vi "ReadAlgoParametersJSON(Override)_General.vi"(7 "Default?":bool, 8 "error in":errorcluster, 9 "Variant?":bool, 10 "Read Edit Tolerance \nOverride JSON":path=path "F:/User Interface Testbench/Configuration file/Zengage System JSON UI.json", 11 "Algo Default JSON":variant) -> (0 "error out":errorcluster, 2 "data":T1, 3 "Algorithm parameters\noverride":T2)   [LabVIEW 2019, in "ZenGage v3.0 UI.lvclass"]
uses:
  ZenGage v3.0 UI.lvclass
  Type Definitions/JSON Read/Algoparameters_default.ctl
panel:
  out "Error Message":string
  out "VCluster\n out":variant
types:
  T1 = cluster{"AlgoParameters":cluster{"PartsList":cluster{"Name":string, "ImageStreams":cluster{"ThreadName":string, "RackEnable":bool, "ThreadId":dbl, "RackId":dbl, "DifferenceParameter":dbl, "SplitCameraIDs":i32[], "ImagingViews":cluster{"ViewName":string, "ViewEnable":bool, "ImageID":dbl, "CameraID":dbl, "CalibrationFilePath":string, "CalibImageFormat":string, "ReferenceCoordSystem":cluster{"Method":cluster{"Algo":string, "BaseReference":cluster{"OriginX":dbl, "OriginY":dbl, "Angle":dbl, "AxisReference":dbl}}, "ROI":cluster{"ROI":cluster{"Left":dbl, "Top":dbl, "Right":dbl, "Bottom":dbl, "Rotation":dbl}, "EdgeOptions":cluster{"EdgePolarity":dbl, "KernelSize":dbl, "Width":dbl, "MinimumEdgeStrength":dbl, "InterpolationType":dbl, "DataProcessingMethod":dbl}, "LineOptions":cluster{"NumberofLines":dbl, "Type":dbl, "MinScore":dbl, "MaxScore":dbl, "Orientation":dbl, "AngleRange":dbl, "AngleTolerance":dbl, "StepSize":dbl, "MinSNR":dbl, "MinPoints":dbl, "HoughIterations":dbl}, "Process":dbl, "StepSize":dbl, "SearchDirection":dbl, "CircleEdgeOptions":cluster{"SearchDirection":dbl, "EdgeOptions":cluster{"EdgePolarity":dbl, "KernelSize":dbl, "Width":dbl, "MinimumEdgeStrength":dbl, "InterpolationType":dbl, "DataProcessingMethod":dbl}}, "CircleFitOptions":cluster{"Process":dbl, "StepSize":dbl, "MAxPixelRadius":dbl}, "CircleSearchDirection":dbl, "CurveParameters":cluster{"ExtractionMode":dbl, "EdgeThreshold":dbl, "EdgeFilterSize":dbl, "MinLength":dbl, "RowSearchStepSize":dbl, "ColSearchStepSize":dbl, "MaxEndpointGap":dbl, "Closed":bool, "Subpixel":bool}, "MinimumMatchScore":dbl, "CircleDescriptor":cluster{"MinRadius":dbl, "MaxRadius":dbl}, "EllipseDescriptor":cluster{"MinMajorRadius":dbl, "MaxMajorRadius":dbl, "MinMinorRadius":dbl, "MaxMinorRadius":dbl}, "ParallelLines":cluster{"First":dbl, "Second":dbl, "Third":dbl}}[], "Name":string, "OverlayOptions":cluster{"OverlayEnable":bool, "OverlayText":string, "OverlayCoords":i32[], "OverlayAngle":dbl, "OverlayTextSize":dbl, "OverlayTextColor":string, "OverlayROI":bool, "OverlayRakeLine":bool, "OverlayPoints":bool}}, "CameraAngle":i32[]}[]}[], "Measurements":cluster{"RackID":dbl, "ImageID":dbl, "CameraID":dbl, "MeasurementId":dbl, "Name":string, "AlgoName":string, "Type":string, "MeasurementEnable":bool, "AlgorithmSequence":cluster{"RefernceEdge":cluster{"Enable":bool, "Method":string, "RefROI":cluster{"Left":dbl, "Top":dbl, "Right":dbl, "Bottom":dbl, "Rotation":dbl}, "EdgeOptions":cluster{"EdgePoarity":dbl, "KernelSize":dbl, "Width":dbl, "MinimumEdgeStrength":dbl, "InterpolationType":dbl, "DataProcessingMethod":dbl}, "LineOptions":cluster{"NumberofLines":dbl, "Type":dbl, "MinScore":dbl, "MaxScore":dbl, "Orientation":dbl, "AngleRange":dbl, "AngleTolerance":dbl, "StepSize":dbl, "MinSNR":dbl, "MinPoints":dbl, "HoughIterations":dbl}, "SearchDirection":dbl}, "Measurement":cluster{"ROI1":cluster{"Enable":bool, "ROI":cluster{"Left":dbl, "Top":dbl, "Right":dbl, "Bottom":dbl, "Rotation":dbl}, "EdgeOptions":cluster{"EdgePoarity":dbl, "KernelSize":dbl, "Width":dbl, "MinimumEdgeStrength":dbl, "InterpolationType":dbl, "DataProcessingMethod":dbl}, "LineOptions":cluster{"NumberofLines":dbl, "Type":dbl, "MinScore":dbl, "MaxScore":dbl, "Orientation":dbl, "AngleRange":dbl, "AngleTolerance":dbl, "StepSize":dbl, "MinSNR":dbl, "MinPoints":dbl, "HoughIterations":dbl}, "Process":dbl, "StepSize":dbl, "SearchDirection":dbl, "CircleEdgeOptions":cluster{"SearchDirection":dbl, "EdgeOptions":cluster{"EdgePoarity":dbl, "KernelSize":dbl, "Width":dbl, "MinimumEdgeStrength":dbl, "InterpolationType":dbl, "DataProcessingMethod":dbl}}, "CircleFitOptions":cluster{"Process":dbl, "StepSize":dbl, "MAxPixelRadius":dbl}, "CircleSearchDirection":dbl, "CurveParameters":cluster{"ExtractionMode":dbl, "EdgeThreshold":dbl, "EdgeFilterSize":dbl, "MinLength":dbl, "RowSearchStepSize":dbl, "ColSearchStepSize":dbl, "MaxEndpointGap":dbl, "Closed":bool, "Subpixel":bool}, "MinimumMatchScore":dbl, "CircleDescriptor":cluster{"MinRadius":dbl, "MaxRadius":dbl}, "EllipseDescriptor":cluster{"MinMajorRadius":dbl, "MaxMajorRadius":dbl, "MinMinorRadius":dbl, "MaxMinorRadius":dbl}}, "ROI2":cluster{"Enable":bool, "ROI":cluster{"Left":dbl, "Top":dbl, "Right":dbl, "Bottom":dbl, "Rotation":dbl}, "EdgeOptions":cluster{"EdgePoarity":dbl, "KernelSize":dbl, "Width":dbl, "MinimumEdgeStrength":dbl, "InterpolationType":dbl, "DataProcessingMethod":dbl}, "LineOptions":cluster{"NumberofLines":dbl, "Type":dbl, "MinScore":dbl, "MaxScore":dbl, "Orientation":dbl, "AngleRange":dbl, "AngleTolerance":dbl, "StepSize":dbl, "MinSNR":dbl, "MinPoints":dbl, "HoughIterations":dbl}, "Process":dbl, "StepSize":dbl, "SearchDirection":dbl, "CircleEdgeOptions":cluster{"SearchDirection":dbl, "EdgeOptions":cluster{"EdgePoarity":dbl, "KernelSize":dbl, "Width":dbl, "MinimumEdgeStrength":dbl, "InterpolationType":dbl, "DataProcessingMethod":dbl}}, "CircleFitOptions":cluster{"Process":dbl, "StepSize":dbl, "MAxPixelRadius":dbl}, "CircleSearchDirection":dbl, "CurveParameters":cluster{"ExtractionMode":dbl, "EdgeThreshold":dbl, "EdgeFilterSize":dbl, "MinLength":dbl, "RowSearchStepSize":dbl, "ColSearchStepSize":dbl, "MaxEndpointGap":dbl, "Closed":bool, "Subpixel":bool}, "MinimumMatchScore":dbl, "CircleDescriptor":cluster{"MinRadius":dbl, "MaxRadius":dbl}, "EllipseDescriptor":cluster{"MinMajorRadius":dbl, "MaxMajorRadius":dbl, "MinMinorRadius":dbl, "MaxMinorRadius":dbl}}}}, "MathExpression":cluster{"Algorithm":string, "MathExpression":string, "ResultVariable":string}, "MathCorrectionParameters":cluster{"Radius":dbl, "CurlGap":dbl, "Thickness":dbl, "MeasurementIndices":i32[], "MathAlgoName":string, "MathAlgoFormula":string, "CorrectionForAngle":i32[], "NumericAray":i32[], "StringArray":string[]}, "ResultVariableCluster":cluster{"RVName":string, "RVSequence":string, "RVIndex":dbl, "RVID":dbl, "RVValue":dbl}, "CalibrationCoefficients":cluster{"A1":dbl, "A2":dbl, "A3":dbl}, "UserCalibCoefficients":cluster{"UserCorrectionLinearityCoeff":dbl, "UserCorrectionBiasCoeff":dbl}, "SpecValues":cluster{"LCL":dbl, "UCL":dbl, "LSL":dbl, "USL":dbl, "NominalValue":dbl}, "OverlayOptions":cluster{"OverlayEnable":bool, "OverlayText":string, "OverlayCoords":i32[], "OverlayAngle":dbl, "OverlayTextSize":dbl, "OverlayTextColor":string, "OverlayROI":bool, "OverlayRakeLine":bool, "OverlayPoints":bool}, "DatalogEnable":bool, "DisplayIcon":string}[]}[], "AlgoDefaultParameters":cluster{"AlgoName":string, "Enable":bool, "AlgorithmSequenceDefault":cluster{"RefernceEdgeDefault":cluster{"Method":string, "RefROI":cluster{"Left":dbl, "Top":dbl, "Right":dbl, "Bottom":dbl, "Rotation":dbl}, "EdgeOptions":cluster{"EdgePoarity":dbl, "KernelSize":dbl, "Width":dbl, "MinimumEdgeStrength":dbl, "InterpolationType":dbl, "DataProcessingMethod":dbl}, "LineOptions":cluster{"NumberofLines":dbl, "Type":dbl, "MinScore":dbl, "MaxScore":dbl, "Orientation":dbl, "AngleRange":dbl, "AngleTolerance":dbl, "StepSize":dbl, "MinSNR":dbl, "MinPoints":dbl, "HoughIterations":dbl}, "SearchDirection":dbl}, "MeasurementDefault":cluster{"ROI1":cluster{"ROI":cluster{"Left":dbl, "Top":dbl, "Right":dbl, "Bottom":dbl, "Rotation":dbl}, "EdgeOptions":cluster{"EdgePoarity":dbl, "KernelSize":dbl, "Width":dbl, "MinimumEdgeStrength":dbl, "InterpolationType":dbl, "DataProcessingMethod":dbl}, "LineOptions":cluster{"NumberofLines":dbl, "Type":dbl, "MinScore":dbl, "MaxScore":dbl, "Orientation":dbl, "AngleRange":dbl, "AngleTolerance":dbl, "StepSize":dbl, "MinSNR":dbl, "MinPoints":dbl, "HoughIterations":dbl}, "Process":dbl, "StepSize":dbl, "SearchDirection":dbl, "CircleEdgeOptions":cluster{"SearchDirection":dbl, "EdgeOptions":cluster{"EdgePoarity":dbl, "KernelSize":dbl, "Width":dbl, "MinimumEdgeStrength":dbl, "InterpolationType":dbl, "DataProcessingMethod":dbl}}, "CircleFitOptions":cluster{"Process":dbl, "StepSize":dbl, "MAxPixelRadius":dbl}, "CircleSearchDirection":dbl, "CurveParameters":cluster{"ExtractionMode":dbl, "EdgeThreshold":dbl, "EdgeFilterSize":dbl, "MinLength":dbl, "RowSearchStepSize":dbl, "ColSearchStepSize":dbl, "MaxEndpointGap":dbl, "Closed":dbl, "Subpixel":dbl}, "MinimumMatchScore":dbl, "CircleDescriptor":cluster{"MinRadius":dbl, "MaxRadius":dbl}, "EllipseDescriptor":cluster{"MinMajorRadius":dbl, "MaxMajorRadius":dbl, "MinMinorRadius":dbl, "MaxMinorRadius":dbl}, "OverlayOptions":cluster{"OverlayEnable":bool, "OverlayText":string, "OverlayCoords":i32[], "OverlayAngle":dbl, "OverlayTextSize":dbl, "OverlayTextColor":string}, "ResultVariable":string}, "ROI2":cluster{"ROI":cluster{"Left":dbl, "Top":dbl, "Right":dbl, "Bottom":dbl, "Rotation":dbl}, "EdgeOptions":cluster{"EdgePoarity":dbl, "KernelSize":dbl, "Width":dbl, "MinimumEdgeStrength":dbl, "InterpolationType":dbl, "DataProcessingMethod":dbl}, "LineOptions":cluster{"NumberofLines":dbl, "Type":dbl, "MinScore":dbl, "MaxScore":dbl, "Orientation":dbl, "AngleRange":dbl, "AngleTolerance":dbl, "StepSize":dbl, "MinSNR":dbl, "MinPoints":dbl, "HoughIterations":dbl}, "Process":dbl, "StepSize":dbl, "SearchDirection":dbl, "CircleEdgeOptions":cluster{"SearchDirection":dbl, "EdgeOptions":cluster{"EdgePoarity":dbl, "KernelSize":dbl, "Width":dbl, "MinimumEdgeStrength":dbl, "InterpolationType":dbl, "DataProcessingMethod":dbl}}, "CircleFitOptions":cluster{"Process":dbl, "StepSize":dbl, "MaxPixelRadius":dbl}, "CircleSearchDirection":dbl, "CurveParameters":cluster{"ExtractionMode":dbl, "EdgeThreshold":dbl, "EdgeFilterSize":dbl, "MinLength":dbl, "RowSearchStepSize":dbl, "ColSearchStepSize":dbl, "MaxEndpointGap":dbl, "Closed":dbl, "Subpixel":dbl}, "MinimumMatchScore":dbl, "CircleDescriptor":cluster{"MinRadius":dbl, "MaxRadius":dbl}, "EllipseDescriptor":cluster{"MinMajorRadius":dbl, "MaxMajorRadius":dbl, "MinMinorRadius":dbl, "MaxMinorRadius":dbl}, "OverlayOptions":cluster{"OverlayEnable":bool, "OverlayText":string, "OverlayCoords":i32[], "OverlayAngle":dbl, "OverlayTextSize":dbl, "OverlayTextColor":string}, "ResultVariable":string}}, "MathExpressionDefault":cluster{"Algorithm":string, "MathExpression":string, "ResultVariable":string}}, "CalibrationCoefficients":cluster{"A1":dbl, "A2":dbl, "A3":dbl}, "UserCalibCoefficients":cluster{"UserCorrectionBiasCoeff":dbl, "UserCorrectionLinearityCoeff":dbl}, "OverlayOptions":cluster{"OverlayEnable":bool, "OverlayText":string, "OverlayCoords":i32[], "OverlayAngle":dbl, "OverlayTextSize":dbl, "OverlayTextColor":string}, "DatalogEnable":bool, "DisplayIcon":string}}}
  T2 = typedef "ZenGage v3.0 UI.lvclass/Algoparameters_default.ctl" = cluster{"AlgoParameters":cluster{"PartsList":cluster{"Name":string, "ImageStreams":cluster{"ThreadName":string, "RackEnable":bool, "ThreadId":dbl, "RackId":dbl, "DifferenceParameter":dbl, "SplitCameraIDs":i32[], "ImagingViews":cluster{"ViewName":string, "ViewEnable":bool, "ImageID":dbl, "CameraID":dbl, "CalibrationFilePath":string, "CalibImageFormat":string, "ReferenceCoordSystem":cluster{"Method":cluster{"Algo":string, "BaseReference":cluster{"OriginX":dbl, "OriginY":dbl, "Angle":dbl, "AxisReference":dbl}}, "ROI":cluster{"ROI":cluster{"Left":dbl, "Top":dbl, "Right":dbl, "Bottom":dbl, "Rotation":dbl}, "EdgeOptions":cluster{"EdgePolarity":dbl, "KernelSize":dbl, "Width":dbl, "MinimumEdgeStrength":dbl, "InterpolationType":dbl, "DataProcessingMethod":dbl}, "LineOptions":cluster{"NumberofLines":dbl, "Type":dbl, "MinScore":dbl, "MaxScore":dbl, "Orientation":dbl, "AngleRange":dbl, "AngleTolerance":dbl, "StepSize":dbl, "MinSNR":dbl, "MinPoints":dbl, "HoughIterations":dbl}, "Process":dbl, "StepSize":dbl, "SearchDirection":dbl, "CircleEdgeOptions":cluster{"SearchDirection":dbl, "EdgeOptions":cluster{"EdgePolarity":dbl, "KernelSize":dbl, "Width":dbl, "MinimumEdgeStrength":dbl, "InterpolationType":dbl, "DataProcessingMethod":dbl}}, "CircleFitOptions":cluster{"Process":dbl, "StepSize":dbl, "MAxPixelRadius":dbl}, "CircleSearchDirection":dbl, "CurveParameters":cluster{"ExtractionMode":dbl, "EdgeThreshold":dbl, "EdgeFilterSize":dbl, "MinLength":dbl, "RowSearchStepSize":dbl, "ColSearchStepSize":dbl, "MaxEndpointGap":dbl, "Closed":bool, "Subpixel":bool}, "MinimumMatchScore":dbl, "CircleDescriptor":cluster{"MinRadius":dbl, "MaxRadius":dbl}, "EllipseDescriptor":cluster{"MinMajorRadius":dbl, "MaxMajorRadius":dbl, "MinMinorRadius":dbl, "MaxMinorRadius":dbl}, "ParallelLines":cluster{"First":dbl, "Second":dbl, "Third":dbl}}[], "Name":string, "OverlayOptions":cluster{"OverlayEnable":bool, "OverlayText":string, "OverlayCoords":i32[], "OverlayAngle":dbl, "OverlayTextSize":dbl, "OverlayTextColor":string, "OverlayROI":bool, "OverlayRakeLine":bool, "OverlayPoints":bool}}}[]}[], "Measurements":cluster{"RackID":dbl, "ImageID":dbl, "CameraID":dbl, "MeasurementId":dbl, "Name":string, "AlgoName":string, "Type":string, "MeasurementEnable":bool, "AlgorithmSequence":cluster{"RefernceEdge":cluster{"Enable":bool, "Method":string, "RefROI":cluster{"Left":dbl, "Top":dbl, "Right":dbl, "Bottom":dbl, "Rotation":dbl}, "EdgeOptions":cluster{"EdgePoarity":dbl, "KernelSize":dbl, "Width":dbl, "MinimumEdgeStrength":dbl, "InterpolationType":dbl, "DataProcessingMethod":dbl}, "LineOptions":cluster{"NumberofLines":dbl, "Type":dbl, "MinScore":dbl, "MaxScore":dbl, "Orientation":dbl, "AngleRange":dbl, "AngleTolerance":dbl, "StepSize":dbl, "MinSNR":dbl, "MinPoints":dbl, "HoughIterations":dbl}, "SearchDirection":dbl}, "Measurement":cluster{"ROI1":cluster{"Enable":bool, "ROI":cluster{"Left":dbl, "Top":dbl, "Right":dbl, "Bottom":dbl, "Rotation":dbl}, "EdgeOptions":cluster{"EdgePoarity":dbl, "KernelSize":dbl, "Width":dbl, "MinimumEdgeStrength":dbl, "InterpolationType":dbl, "DataProcessingMethod":dbl}, "LineOptions":cluster{"NumberofLines":dbl, "Type":dbl, "MinScore":dbl, "MaxScore":dbl, "Orientation":dbl, "AngleRange":dbl, "AngleTolerance":dbl, "StepSize":dbl, "MinSNR":dbl, "MinPoints":dbl, "HoughIterations":dbl}, "Process":dbl, "StepSize":dbl, "SearchDirection":dbl, "CircleEdgeOptions":cluster{"SearchDirection":dbl, "EdgeOptions":cluster{"EdgePoarity":dbl, "KernelSize":dbl, "Width":dbl, "MinimumEdgeStrength":dbl, "InterpolationType":dbl, "DataProcessingMethod":dbl}}, "CircleFitOptions":cluster{"Process":dbl, "StepSize":dbl, "MAxPixelRadius":dbl}, "CircleSearchDirection":dbl, "CurveParameters":cluster{"ExtractionMode":dbl, "EdgeThreshold":dbl, "EdgeFilterSize":dbl, "MinLength":dbl, "RowSearchStepSize":dbl, "ColSearchStepSize":dbl, "MaxEndpointGap":dbl, "Closed":bool, "Subpixel":bool}, "MinimumMatchScore":dbl, "CircleDescriptor":cluster{"MinRadius":dbl, "MaxRadius":dbl}, "EllipseDescriptor":cluster{"MinMajorRadius":dbl, "MaxMajorRadius":dbl, "MinMinorRadius":dbl, "MaxMinorRadius":dbl}}, "ROI2":cluster{"Enable":bool, "ROI":cluster{"Left":dbl, "Top":dbl, "Right":dbl, "Bottom":dbl, "Rotation":dbl}, "EdgeOptions":cluster{"EdgePoarity":dbl, "KernelSize":dbl, "Width":dbl, "MinimumEdgeStrength":dbl, "InterpolationType":dbl, "DataProcessingMethod":dbl}, "LineOptions":cluster{"NumberofLines":dbl, "Type":dbl, "MinScore":dbl, "MaxScore":dbl, "Orientation":dbl, "AngleRange":dbl, "AngleTolerance":dbl, "StepSize":dbl, "MinSNR":dbl, "MinPoints":dbl, "HoughIterations":dbl}, "Process":dbl, "StepSize":dbl, "SearchDirection":dbl, "CircleEdgeOptions":cluster{"SearchDirection":dbl, "EdgeOptions":cluster{"EdgePoarity":dbl, "KernelSize":dbl, "Width":dbl, "MinimumEdgeStrength":dbl, "InterpolationType":dbl, "DataProcessingMethod":dbl}}, "CircleFitOptions":cluster{"Process":dbl, "StepSize":dbl, "MAxPixelRadius":dbl}, "CircleSearchDirection":dbl, "CurveParameters":cluster{"ExtractionMode":dbl, "EdgeThreshold":dbl, "EdgeFilterSize":dbl, "MinLength":dbl, "RowSearchStepSize":dbl, "ColSearchStepSize":dbl, "MaxEndpointGap":dbl, "Closed":bool, "Subpixel":bool}, "MinimumMatchScore":dbl, "CircleDescriptor":cluster{"MinRadius":dbl, "MaxRadius":dbl}, "EllipseDescriptor":cluster{"MinMajorRadius":dbl, "MaxMajorRadius":dbl, "MinMinorRadius":dbl, "MaxMinorRadius":dbl}}}}, "MathExpression":cluster{"Algorithm":string, "MathExpression":string, "ResultVariable":string}, "ResultVariableCluster":cluster{"RVName":string, "RVSequence":string, "RVIndex":dbl, "RVID":dbl, "RVValue":dbl}, "CalibrationCoefficients":cluster{"A1":dbl, "A2":dbl, "A3":dbl}, "UserCalibCoefficients":cluster{"UserCorrectionLinearityCoeff":dbl, "UserCorrectionBiasCoeff":dbl}, "SpecValues":cluster{"LCL":dbl, "UCL":dbl, "LSL":dbl, "USL":dbl, "NominalValue":dbl}, "OverlayOptions":cluster{"OverlayEnable":bool, "OverlayText":string, "OverlayCoords":i32[], "OverlayAngle":dbl, "OverlayTextSize":dbl, "OverlayTextColor":string, "OverlayROI":bool, "OverlayRakeLine":bool, "OverlayPoints":bool}, "DatalogEnable":bool, "DisplayIcon":string}[]}[], "AlgoDefaultParameters":cluster{"AlgoName":string, "Enable":bool, "AlgorithmSequenceDefault":cluster{"RefernceEdgeDefault":cluster{"Method":string, "RefROI":cluster{"Left":dbl, "Top":dbl, "Right":dbl, "Bottom":dbl, "Rotation":dbl}, "EdgeOptions":cluster{"EdgePoarity":dbl, "KernelSize":dbl, "Width":dbl, "MinimumEdgeStrength":dbl, "InterpolationType":dbl, "DataProcessingMethod":dbl}, "LineOptions":cluster{"NumberofLines":dbl, "Type":dbl, "MinScore":dbl, "MaxScore":dbl, "Orientation":dbl, "AngleRange":dbl, "AngleTolerance":dbl, "StepSize":dbl, "MinSNR":dbl, "MinPoints":dbl, "HoughIterations":dbl}, "SearchDirection":dbl}, "MeasurementDefault":cluster{"ROI1":cluster{"ROI":cluster{"Left":dbl, "Top":dbl, "Right":dbl, "Bottom":dbl, "Rotation":dbl}, "EdgeOptions":cluster{"EdgePoarity":dbl, "KernelSize":dbl, "Width":dbl, "MinimumEdgeStrength":dbl, "InterpolationType":dbl, "DataProcessingMethod":dbl}, "LineOptions":cluster{"NumberofLines":dbl, "Type":dbl, "MinScore":dbl, "MaxScore":dbl, "Orientation":dbl, "AngleRange":dbl, "AngleTolerance":dbl, "StepSize":dbl, "MinSNR":dbl, "MinPoints":dbl, "HoughIterations":dbl}, "Process":dbl, "StepSize":dbl, "SearchDirection":dbl, "CircleEdgeOptions":cluster{"SearchDirection":dbl, "EdgeOptions":cluster{"EdgePoarity":dbl, "KernelSize":dbl, "Width":dbl, "MinimumEdgeStrength":dbl, "InterpolationType":dbl, "DataProcessingMethod":dbl}}, "CircleFitOptions":cluster{"Process":dbl, "StepSize":dbl, "MAxPixelRadius":dbl}, "CircleSearchDirection":dbl, "CurveParameters":cluster{"ExtractionMode":dbl, "EdgeThreshold":dbl, "EdgeFilterSize":dbl, "MinLength":dbl, "RowSearchStepSize":dbl, "ColSearchStepSize":dbl, "MaxEndpointGap":dbl, "Closed":dbl, "Subpixel":dbl}, "MinimumMatchScore":dbl, "CircleDescriptor":cluster{"MinRadius":dbl, "MaxRadius":dbl}, "EllipseDescriptor":cluster{"MinMajorRadius":dbl, "MaxMajorRadius":dbl, "MinMinorRadius":dbl, "MaxMinorRadius":dbl}, "OverlayOptions":cluster{"OverlayEnable":bool, "OverlayText":string, "OverlayCoords":i32[], "OverlayAngle":dbl, "OverlayTextSize":dbl, "OverlayTextColor":string}, "ResultVariable":string}, "ROI2":cluster{"ROI":cluster{"Left":dbl, "Top":dbl, "Right":dbl, "Bottom":dbl, "Rotation":dbl}, "EdgeOptions":cluster{"EdgePoarity":dbl, "KernelSize":dbl, "Width":dbl, "MinimumEdgeStrength":dbl, "InterpolationType":dbl, "DataProcessingMethod":dbl}, "LineOptions":cluster{"NumberofLines":dbl, "Type":dbl, "MinScore":dbl, "MaxScore":dbl, "Orientation":dbl, "AngleRange":dbl, "AngleTolerance":dbl, "StepSize":dbl, "MinSNR":dbl, "MinPoints":dbl, "HoughIterations":dbl}, "Process":dbl, "StepSize":dbl, "SearchDirection":dbl, "CircleEdgeOptions":cluster{"SearchDirection":dbl, "EdgeOptions":cluster{"EdgePoarity":dbl, "KernelSize":dbl, "Width":dbl, "MinimumEdgeStrength":dbl, "InterpolationType":dbl, "DataProcessingMethod":dbl}}, "CircleFitOptions":cluster{"Process":dbl, "StepSize":dbl, "MaxPixelRadius":dbl}, "CircleSearchDirection":dbl, "CurveParameters":cluster{"ExtractionMode":dbl, "EdgeThreshold":dbl, "EdgeFilterSize":dbl, "MinLength":dbl, "RowSearchStepSize":dbl, "ColSearchStepSize":dbl, "MaxEndpointGap":dbl, "Closed":dbl, "Subpixel":dbl}, "MinimumMatchScore":dbl, "CircleDescriptor":cluster{"MinRadius":dbl, "MaxRadius":dbl}, "EllipseDescriptor":cluster{"MinMajorRadius":dbl, "MaxMajorRadius":dbl, "MinMinorRadius":dbl, "MaxMinorRadius":dbl}, "OverlayOptions":cluster{"OverlayEnable":bool, "OverlayText":string, "OverlayCoords":i32[], "OverlayAngle":dbl, "OverlayTextSize":dbl, "OverlayTextColor":string}, "ResultVariable":string}}, "MathExpressionDefault":cluster{"Algorithm":string, "MathExpression":string, "ResultVariable":string}}, "CalibrationCoefficients":cluster{"A1":dbl, "A2":dbl, "A3":dbl}, "UserCalibCoefficients":cluster{"UserCorrectionBiasCoeff":dbl, "UserCorrectionLinearityCoeff":dbl}, "OverlayOptions":cluster{"OverlayEnable":bool, "OverlayText":string, "OverlayCoords":i32[], "OverlayAngle":dbl, "OverlayTextSize":dbl, "OverlayTextColor":string}, "DatalogEnable":bool, "DisplayIcon":string}}}
  T3 = cluster{"SpecificationVersion":string, "CompatibleSoftwareVersions":string[], "AlgoParameters":cluster{"PartsList":cluster{"Name":string, "ImageStreams":cluster{"ThreadName":string, "RackEnable":bool, "ThreadId":dbl, "RackId":dbl, "DifferenceParameter":dbl, "SplitCameraIDs":i32[], "ImagingViews":cluster{"ViewName":string, "ViewEnable":bool, "ImageID":dbl, "CameraID":dbl, "CalibrationFilePath":string, "CalibImageFormat":string, "ReferenceCoordSystem":cluster{"Method":cluster{"Algo":string, "BaseReference":cluster{"OriginX":dbl, "OriginY":dbl, "Angle":dbl, "AxisReference":dbl}}, "ROI":cluster{"ROI":cluster{"Left":dbl, "Top":dbl, "Right":dbl, "Bottom":dbl, "Rotation":dbl}, "EdgeOptions":cluster{"EdgePolarity":dbl, "KernelSize":dbl, "Width":dbl, "MinimumEdgeStrength":dbl, "InterpolationType":dbl, "DataProcessingMethod":dbl}, "LineOptions":cluster{"NumberofLines":dbl, "Type":dbl, "MinScore":dbl, "MaxScore":dbl, "Orientation":dbl, "AngleRange":dbl, "AngleTolerance":dbl, "StepSize":dbl, "MinSNR":dbl, "MinPoints":dbl, "HoughIterations":dbl}, "Process":dbl, "StepSize":dbl, "SearchDirection":dbl, "CircleEdgeOptions":cluster{"SearchDirection":dbl, "EdgeOptions":cluster{"EdgePolarity":dbl, "KernelSize":dbl, "Width":dbl, "MinimumEdgeStrength":dbl, "InterpolationType":dbl, "DataProcessingMethod":dbl}}, "CircleFitOptions":cluster{"Process":dbl, "StepSize":dbl, "MAxPixelRadius":dbl}, "CircleSearchDirection":dbl, "CurveParameters":cluster{"ExtractionMode":dbl, "EdgeThreshold":dbl, "EdgeFilterSize":dbl, "MinLength":dbl, "RowSearchStepSize":dbl, "ColSearchStepSize":dbl, "MaxEndpointGap":dbl, "Closed":bool, "Subpixel":bool}, "MinimumMatchScore":dbl, "CircleDescriptor":cluster{"MinRadius":dbl, "MaxRadius":dbl}, "EllipseDescriptor":cluster{"MinMajorRadius":dbl, "MaxMajorRadius":dbl, "MinMinorRadius":dbl, "MaxMinorRadius":dbl}, "ParallelLines":cluster{"First":dbl, "Second":dbl, "Third":dbl}}[], "Name":string, "OverlayOptions":cluster{"OverlayEnable":bool, "OverlayText":string, "OverlayCoords":i32[], "OverlayAngle":dbl, "OverlayTextSize":dbl, "OverlayTextColor":string, "OverlayROI":bool, "OverlayRakeLine":bool, "OverlayPoints":bool}}, "CameraAngle":i32[]}[]}[], "Measurements":cluster{"RackID":dbl, "ImageID":dbl, "CameraID":dbl, "MeasurementId":dbl, "Name":string, "AlgoName":string, "Type":string, "MeasurementEnable":bool, "AlgorithmSequence":cluster{"RefernceEdge":cluster{"Enable":bool, "Method":string, "RefROI":cluster{"Left":dbl, "Top":dbl, "Right":dbl, "Bottom":dbl, "Rotation":dbl}, "EdgeOptions":cluster{"EdgePoarity":dbl, "KernelSize":dbl, "Width":dbl, "MinimumEdgeStrength":dbl, "InterpolationType":dbl, "DataProcessingMethod":dbl}, "LineOptions":cluster{"NumberofLines":dbl, "Type":dbl, "MinScore":dbl, "MaxScore":dbl, "Orientation":dbl, "AngleRange":dbl, "AngleTolerance":dbl, "StepSize":dbl, "MinSNR":dbl, "MinPoints":dbl, "HoughIterations":dbl}, "SearchDirection":dbl}, "Measurement":cluster{"ROI1":cluster{"Enable":bool, "ROI":cluster{"Left":dbl, "Top":dbl, "Right":dbl, "Bottom":dbl, "Rotation":dbl}, "EdgeOptions":cluster{"EdgePoarity":dbl, "KernelSize":dbl, "Width":dbl, "MinimumEdgeStrength":dbl, "InterpolationType":dbl, "DataProcessingMethod":dbl}, "LineOptions":cluster{"NumberofLines":dbl, "Type":dbl, "MinScore":dbl, "MaxScore":dbl, "Orientation":dbl, "AngleRange":dbl, "AngleTolerance":dbl, "StepSize":dbl, "MinSNR":dbl, "MinPoints":dbl, "HoughIterations":dbl}, "Process":dbl, "StepSize":dbl, "SearchDirection":dbl, "CircleEdgeOptions":cluster{"SearchDirection":dbl, "EdgeOptions":cluster{"EdgePoarity":dbl, "KernelSize":dbl, "Width":dbl, "MinimumEdgeStrength":dbl, "InterpolationType":dbl, "DataProcessingMethod":dbl}}, "CircleFitOptions":cluster{"Process":dbl, "StepSize":dbl, "MAxPixelRadius":dbl}, "CircleSearchDirection":dbl, "CurveParameters":cluster{"ExtractionMode":dbl, "EdgeThreshold":dbl, "EdgeFilterSize":dbl, "MinLength":dbl, "RowSearchStepSize":dbl, "ColSearchStepSize":dbl, "MaxEndpointGap":dbl, "Closed":bool, "Subpixel":bool}, "MinimumMatchScore":dbl, "CircleDescriptor":cluster{"MinRadius":dbl, "MaxRadius":dbl}, "EllipseDescriptor":cluster{"MinMajorRadius":dbl, "MaxMajorRadius":dbl, "MinMinorRadius":dbl, "MaxMinorRadius":dbl}}, "ROI2":cluster{"Enable":bool, "ROI":cluster{"Left":dbl, "Top":dbl, "Right":dbl, "Bottom":dbl, "Rotation":dbl}, "EdgeOptions":cluster{"EdgePoarity":dbl, "KernelSize":dbl, "Width":dbl, "MinimumEdgeStrength":dbl, "InterpolationType":dbl, "DataProcessingMethod":dbl}, "LineOptions":cluster{"NumberofLines":dbl, "Type":dbl, "MinScore":dbl, "MaxScore":dbl, "Orientation":dbl, "AngleRange":dbl, "AngleTolerance":dbl, "StepSize":dbl, "MinSNR":dbl, "MinPoints":dbl, "HoughIterations":dbl}, "Process":dbl, "StepSize":dbl, "SearchDirection":dbl, "CircleEdgeOptions":cluster{"SearchDirection":dbl, "EdgeOptions":cluster{"EdgePoarity":dbl, "KernelSize":dbl, "Width":dbl, "MinimumEdgeStrength":dbl, "InterpolationType":dbl, "DataProcessingMethod":dbl}}, "CircleFitOptions":cluster{"Process":dbl, "StepSize":dbl, "MAxPixelRadius":dbl}, "CircleSearchDirection":dbl, "CurveParameters":cluster{"ExtractionMode":dbl, "EdgeThreshold":dbl, "EdgeFilterSize":dbl, "MinLength":dbl, "RowSearchStepSize":dbl, "ColSearchStepSize":dbl, "MaxEndpointGap":dbl, "Closed":bool, "Subpixel":bool}, "MinimumMatchScore":dbl, "CircleDescriptor":cluster{"MinRadius":dbl, "MaxRadius":dbl}, "EllipseDescriptor":cluster{"MinMajorRadius":dbl, "MaxMajorRadius":dbl, "MinMinorRadius":dbl, "MaxMinorRadius":dbl}}}}, "MathExpression":cluster{"Algorithm":string, "MathExpression":string, "ResultVariable":string}, "MathCorrectionParameters":cluster{"Radius":dbl, "CurlGap":dbl, "Thickness":dbl, "MeasurementIndices":i32[], "MathAlgoName":string, "MathAlgoFormula":string, "CorrectionForAngle":i32[], "NumericAray":i32[], "StringArray":string[]}, "ResultVariableCluster":cluster{"RVName":string, "RVSequence":string, "RVIndex":dbl, "RVID":dbl, "RVValue":dbl}, "CalibrationCoefficients":cluster{"A1":dbl, "A2":dbl, "A3":dbl}, "UserCalibCoefficients":cluster{"UserCorrectionLinearityCoeff":dbl, "UserCorrectionBiasCoeff":dbl}, "SpecValues":cluster{"LCL":dbl, "UCL":dbl, "LSL":dbl, "USL":dbl, "NominalValue":dbl}, "OverlayOptions":cluster{"OverlayEnable":bool, "OverlayText":string, "OverlayCoords":i32[], "OverlayAngle":dbl, "OverlayTextSize":dbl, "OverlayTextColor":string, "OverlayROI":bool, "OverlayRakeLine":bool, "OverlayPoints":bool}, "DatalogEnable":bool, "DisplayIcon":string}[]}[], "AlgoDefaultParameters":cluster{"AlgoName":string, "Enable":bool, "AlgorithmSequenceDefault":cluster{"RefernceEdgeDefault":cluster{"Method":string, "RefROI":cluster{"Left":dbl, "Top":dbl, "Right":dbl, "Bottom":dbl, "Rotation":dbl}, "EdgeOptions":cluster{"EdgePoarity":dbl, "KernelSize":dbl, "Width":dbl, "MinimumEdgeStrength":dbl, "InterpolationType":dbl, "DataProcessingMethod":dbl}, "LineOptions":cluster{"NumberofLines":dbl, "Type":dbl, "MinScore":dbl, "MaxScore":dbl, "Orientation":dbl, "AngleRange":dbl, "AngleTolerance":dbl, "StepSize":dbl, "MinSNR":dbl, "MinPoints":dbl, "HoughIterations":dbl}, "SearchDirection":dbl}, "MeasurementDefault":cluster{"ROI1":cluster{"ROI":cluster{"Left":dbl, "Top":dbl, "Right":dbl, "Bottom":dbl, "Rotation":dbl}, "EdgeOptions":cluster{"EdgePoarity":dbl, "KernelSize":dbl, "Width":dbl, "MinimumEdgeStrength":dbl, "InterpolationType":dbl, "DataProcessingMethod":dbl}, "LineOptions":cluster{"NumberofLines":dbl, "Type":dbl, "MinScore":dbl, "MaxScore":dbl, "Orientation":dbl, "AngleRange":dbl, "AngleTolerance":dbl, "StepSize":dbl, "MinSNR":dbl, "MinPoints":dbl, "HoughIterations":dbl}, "Process":dbl, "StepSize":dbl, "SearchDirection":dbl, "CircleEdgeOptions":cluster{"SearchDirection":dbl, "EdgeOptions":cluster{"EdgePoarity":dbl, "KernelSize":dbl, "Width":dbl, "MinimumEdgeStrength":dbl, "InterpolationType":dbl, "DataProcessingMethod":dbl}}, "CircleFitOptions":cluster{"Process":dbl, "StepSize":dbl, "MAxPixelRadius":dbl}, "CircleSearchDirection":dbl, "CurveParameters":cluster{"ExtractionMode":dbl, "EdgeThreshold":dbl, "EdgeFilterSize":dbl, "MinLength":dbl, "RowSearchStepSize":dbl, "ColSearchStepSize":dbl, "MaxEndpointGap":dbl, "Closed":dbl, "Subpixel":dbl}, "MinimumMatchScore":dbl, "CircleDescriptor":cluster{"MinRadius":dbl, "MaxRadius":dbl}, "EllipseDescriptor":cluster{"MinMajorRadius":dbl, "MaxMajorRadius":dbl, "MinMinorRadius":dbl, "MaxMinorRadius":dbl}, "OverlayOptions":cluster{"OverlayEnable":bool, "OverlayText":string, "OverlayCoords":i32[], "OverlayAngle":dbl, "OverlayTextSize":dbl, "OverlayTextColor":string}, "ResultVariable":string}, "ROI2":cluster{"ROI":cluster{"Left":dbl, "Top":dbl, "Right":dbl, "Bottom":dbl, "Rotation":dbl}, "EdgeOptions":cluster{"EdgePoarity":dbl, "KernelSize":dbl, "Width":dbl, "MinimumEdgeStrength":dbl, "InterpolationType":dbl, "DataProcessingMethod":dbl}, "LineOptions":cluster{"NumberofLines":dbl, "Type":dbl, "MinScore":dbl, "MaxScore":dbl, "Orientation":dbl, "AngleRange":dbl, "AngleTolerance":dbl, "StepSize":dbl, "MinSNR":dbl, "MinPoints":dbl, "HoughIterations":dbl}, "Process":dbl, "StepSize":dbl, "SearchDirection":dbl, "CircleEdgeOptions":cluster{"SearchDirection":dbl, "EdgeOptions":cluster{"EdgePoarity":dbl, "KernelSize":dbl, "Width":dbl, "MinimumEdgeStrength":dbl, "InterpolationType":dbl, "DataProcessingMethod":dbl}}, "CircleFitOptions":cluster{"Process":dbl, "StepSize":dbl, "MaxPixelRadius":dbl}, "CircleSearchDirection":dbl, "CurveParameters":cluster{"ExtractionMode":dbl, "EdgeThreshold":dbl, "EdgeFilterSize":dbl, "MinLength":dbl, "RowSearchStepSize":dbl, "ColSearchStepSize":dbl, "MaxEndpointGap":dbl, "Closed":dbl, "Subpixel":dbl}, "MinimumMatchScore":dbl, "CircleDescriptor":cluster{"MinRadius":dbl, "MaxRadius":dbl}, "EllipseDescriptor":cluster{"MinMajorRadius":dbl, "MaxMajorRadius":dbl, "MinMinorRadius":dbl, "MaxMinorRadius":dbl}, "OverlayOptions":cluster{"OverlayEnable":bool, "OverlayText":string, "OverlayCoords":i32[], "OverlayAngle":dbl, "OverlayTextSize":dbl, "OverlayTextColor":string}, "ResultVariable":string}}, "MathExpressionDefault":cluster{"Algorithm":string, "MathExpression":string, "ResultVariable":string}}, "CalibrationCoefficients":cluster{"A1":dbl, "A2":dbl, "A3":dbl}, "UserCalibCoefficients":cluster{"UserCorrectionBiasCoeff":dbl, "UserCorrectionLinearityCoeff":dbl}, "OverlayOptions":cluster{"OverlayEnable":bool, "OverlayText":string, "OverlayCoords":i32[], "OverlayAngle":dbl, "OverlayTextSize":dbl, "OverlayTextColor":string}, "DatalogEnable":bool, "DisplayIcon":string}}}
  T4 = cluster{"PartsList":cluster{"Name":string, "ImageStreams":cluster{"ThreadName":string, "RackEnable":bool, "ThreadId":dbl, "RackId":dbl, "DifferenceParameter":dbl, "SplitCameraIDs":i32[], "ImagingViews":cluster{"ViewName":string, "ViewEnable":bool, "ImageID":dbl, "CameraID":dbl, "CalibrationFilePath":string, "CalibImageFormat":string, "ReferenceCoordSystem":cluster{"Method":cluster{"Algo":string, "BaseReference":cluster{"OriginX":dbl, "OriginY":dbl, "Angle":dbl, "AxisReference":dbl}}, "ROI":cluster{"ROI":cluster{"Left":dbl, "Top":dbl, "Right":dbl, "Bottom":dbl, "Rotation":dbl}, "EdgeOptions":cluster{"EdgePolarity":dbl, "KernelSize":dbl, "Width":dbl, "MinimumEdgeStrength":dbl, "InterpolationType":dbl, "DataProcessingMethod":dbl}, "LineOptions":cluster{"NumberofLines":dbl, "Type":dbl, "MinScore":dbl, "MaxScore":dbl, "Orientation":dbl, "AngleRange":dbl, "AngleTolerance":dbl, "StepSize":dbl, "MinSNR":dbl, "MinPoints":dbl, "HoughIterations":dbl}, "Process":dbl, "StepSize":dbl, "SearchDirection":dbl, "CircleEdgeOptions":cluster{"SearchDirection":dbl, "EdgeOptions":cluster{"EdgePolarity":dbl, "KernelSize":dbl, "Width":dbl, "MinimumEdgeStrength":dbl, "InterpolationType":dbl, "DataProcessingMethod":dbl}}, "CircleFitOptions":cluster{"Process":dbl, "StepSize":dbl, "MAxPixelRadius":dbl}, "CircleSearchDirection":dbl, "CurveParameters":cluster{"ExtractionMode":dbl, "EdgeThreshold":dbl, "EdgeFilterSize":dbl, "MinLength":dbl, "RowSearchStepSize":dbl, "ColSearchStepSize":dbl, "MaxEndpointGap":dbl, "Closed":bool, "Subpixel":bool}, "MinimumMatchScore":dbl, "CircleDescriptor":cluster{"MinRadius":dbl, "MaxRadius":dbl}, "EllipseDescriptor":cluster{"MinMajorRadius":dbl, "MaxMajorRadius":dbl, "MinMinorRadius":dbl, "MaxMinorRadius":dbl}, "ParallelLines":cluster{"First":dbl, "Second":dbl, "Third":dbl}}[], "Name":string, "OverlayOptions":cluster{"OverlayEnable":bool, "OverlayText":string, "OverlayCoords":i32[], "OverlayAngle":dbl, "OverlayTextSize":dbl, "OverlayTextColor":string, "OverlayROI":bool, "OverlayRakeLine":bool, "OverlayPoints":bool}}, "CameraAngle":i32[]}[]}[], "Measurements":cluster{"RackID":dbl, "ImageID":dbl, "CameraID":dbl, "MeasurementId":dbl, "Name":string, "AlgoName":string, "Type":string, "MeasurementEnable":bool, "AlgorithmSequence":cluster{"RefernceEdge":cluster{"Enable":bool, "Method":string, "RefROI":cluster{"Left":dbl, "Top":dbl, "Right":dbl, "Bottom":dbl, "Rotation":dbl}, "EdgeOptions":cluster{"EdgePoarity":dbl, "KernelSize":dbl, "Width":dbl, "MinimumEdgeStrength":dbl, "InterpolationType":dbl, "DataProcessingMethod":dbl}, "LineOptions":cluster{"NumberofLines":dbl, "Type":dbl, "MinScore":dbl, "MaxScore":dbl, "Orientation":dbl, "AngleRange":dbl, "AngleTolerance":dbl, "StepSize":dbl, "MinSNR":dbl, "MinPoints":dbl, "HoughIterations":dbl}, "SearchDirection":dbl}, "Measurement":cluster{"ROI1":cluster{"Enable":bool, "ROI":cluster{"Left":dbl, "Top":dbl, "Right":dbl, "Bottom":dbl, "Rotation":dbl}, "EdgeOptions":cluster{"EdgePoarity":dbl, "KernelSize":dbl, "Width":dbl, "MinimumEdgeStrength":dbl, "InterpolationType":dbl, "DataProcessingMethod":dbl}, "LineOptions":cluster{"NumberofLines":dbl, "Type":dbl, "MinScore":dbl, "MaxScore":dbl, "Orientation":dbl, "AngleRange":dbl, "AngleTolerance":dbl, "StepSize":dbl, "MinSNR":dbl, "MinPoints":dbl, "HoughIterations":dbl}, "Process":dbl, "StepSize":dbl, "SearchDirection":dbl, "CircleEdgeOptions":cluster{"SearchDirection":dbl, "EdgeOptions":cluster{"EdgePoarity":dbl, "KernelSize":dbl, "Width":dbl, "MinimumEdgeStrength":dbl, "InterpolationType":dbl, "DataProcessingMethod":dbl}}, "CircleFitOptions":cluster{"Process":dbl, "StepSize":dbl, "MAxPixelRadius":dbl}, "CircleSearchDirection":dbl, "CurveParameters":cluster{"ExtractionMode":dbl, "EdgeThreshold":dbl, "EdgeFilterSize":dbl, "MinLength":dbl, "RowSearchStepSize":dbl, "ColSearchStepSize":dbl, "MaxEndpointGap":dbl, "Closed":bool, "Subpixel":bool}, "MinimumMatchScore":dbl, "CircleDescriptor":cluster{"MinRadius":dbl, "MaxRadius":dbl}, "EllipseDescriptor":cluster{"MinMajorRadius":dbl, "MaxMajorRadius":dbl, "MinMinorRadius":dbl, "MaxMinorRadius":dbl}}, "ROI2":cluster{"Enable":bool, "ROI":cluster{"Left":dbl, "Top":dbl, "Right":dbl, "Bottom":dbl, "Rotation":dbl}, "EdgeOptions":cluster{"EdgePoarity":dbl, "KernelSize":dbl, "Width":dbl, "MinimumEdgeStrength":dbl, "InterpolationType":dbl, "DataProcessingMethod":dbl}, "LineOptions":cluster{"NumberofLines":dbl, "Type":dbl, "MinScore":dbl, "MaxScore":dbl, "Orientation":dbl, "AngleRange":dbl, "AngleTolerance":dbl, "StepSize":dbl, "MinSNR":dbl, "MinPoints":dbl, "HoughIterations":dbl}, "Process":dbl, "StepSize":dbl, "SearchDirection":dbl, "CircleEdgeOptions":cluster{"SearchDirection":dbl, "EdgeOptions":cluster{"EdgePoarity":dbl, "KernelSize":dbl, "Width":dbl, "MinimumEdgeStrength":dbl, "InterpolationType":dbl, "DataProcessingMethod":dbl}}, "CircleFitOptions":cluster{"Process":dbl, "StepSize":dbl, "MAxPixelRadius":dbl}, "CircleSearchDirection":dbl, "CurveParameters":cluster{"ExtractionMode":dbl, "EdgeThreshold":dbl, "EdgeFilterSize":dbl, "MinLength":dbl, "RowSearchStepSize":dbl, "ColSearchStepSize":dbl, "MaxEndpointGap":dbl, "Closed":bool, "Subpixel":bool}, "MinimumMatchScore":dbl, "CircleDescriptor":cluster{"MinRadius":dbl, "MaxRadius":dbl}, "EllipseDescriptor":cluster{"MinMajorRadius":dbl, "MaxMajorRadius":dbl, "MinMinorRadius":dbl, "MaxMinorRadius":dbl}}}}, "MathExpression":cluster{"Algorithm":string, "MathExpression":string, "ResultVariable":string}, "MathCorrectionParameters":cluster{"Radius":dbl, "CurlGap":dbl, "Thickness":dbl, "MeasurementIndices":i32[], "MathAlgoName":string, "MathAlgoFormula":string, "CorrectionForAngle":i32[], "NumericAray":i32[], "StringArray":string[]}, "ResultVariableCluster":cluster{"RVName":string, "RVSequence":string, "RVIndex":dbl, "RVID":dbl, "RVValue":dbl}, "CalibrationCoefficients":cluster{"A1":dbl, "A2":dbl, "A3":dbl}, "UserCalibCoefficients":cluster{"UserCorrectionLinearityCoeff":dbl, "UserCorrectionBiasCoeff":dbl}, "SpecValues":cluster{"LCL":dbl, "UCL":dbl, "LSL":dbl, "USL":dbl, "NominalValue":dbl}, "OverlayOptions":cluster{"OverlayEnable":bool, "OverlayText":string, "OverlayCoords":i32[], "OverlayAngle":dbl, "OverlayTextSize":dbl, "OverlayTextColor":string, "OverlayROI":bool, "OverlayRakeLine":bool, "OverlayPoints":bool}, "DatalogEnable":bool, "DisplayIcon":string}[]}[], "AlgoDefaultParameters":cluster{"AlgoName":string, "Enable":bool, "AlgorithmSequenceDefault":cluster{"RefernceEdgeDefault":cluster{"Method":string, "RefROI":cluster{"Left":dbl, "Top":dbl, "Right":dbl, "Bottom":dbl, "Rotation":dbl}, "EdgeOptions":cluster{"EdgePoarity":dbl, "KernelSize":dbl, "Width":dbl, "MinimumEdgeStrength":dbl, "InterpolationType":dbl, "DataProcessingMethod":dbl}, "LineOptions":cluster{"NumberofLines":dbl, "Type":dbl, "MinScore":dbl, "MaxScore":dbl, "Orientation":dbl, "AngleRange":dbl, "AngleTolerance":dbl, "StepSize":dbl, "MinSNR":dbl, "MinPoints":dbl, "HoughIterations":dbl}, "SearchDirection":dbl}, "MeasurementDefault":cluster{"ROI1":cluster{"ROI":cluster{"Left":dbl, "Top":dbl, "Right":dbl, "Bottom":dbl, "Rotation":dbl}, "EdgeOptions":cluster{"EdgePoarity":dbl, "KernelSize":dbl, "Width":dbl, "MinimumEdgeStrength":dbl, "InterpolationType":dbl, "DataProcessingMethod":dbl}, "LineOptions":cluster{"NumberofLines":dbl, "Type":dbl, "MinScore":dbl, "MaxScore":dbl, "Orientation":dbl, "AngleRange":dbl, "AngleTolerance":dbl, "StepSize":dbl, "MinSNR":dbl, "MinPoints":dbl, "HoughIterations":dbl}, "Process":dbl, "StepSize":dbl, "SearchDirection":dbl, "CircleEdgeOptions":cluster{"SearchDirection":dbl, "EdgeOptions":cluster{"EdgePoarity":dbl, "KernelSize":dbl, "Width":dbl, "MinimumEdgeStrength":dbl, "InterpolationType":dbl, "DataProcessingMethod":dbl}}, "CircleFitOptions":cluster{"Process":dbl, "StepSize":dbl, "MAxPixelRadius":dbl}, "CircleSearchDirection":dbl, "CurveParameters":cluster{"ExtractionMode":dbl, "EdgeThreshold":dbl, "EdgeFilterSize":dbl, "MinLength":dbl, "RowSearchStepSize":dbl, "ColSearchStepSize":dbl, "MaxEndpointGap":dbl, "Closed":dbl, "Subpixel":dbl}, "MinimumMatchScore":dbl, "CircleDescriptor":cluster{"MinRadius":dbl, "MaxRadius":dbl}, "EllipseDescriptor":cluster{"MinMajorRadius":dbl, "MaxMajorRadius":dbl, "MinMinorRadius":dbl, "MaxMinorRadius":dbl}, "OverlayOptions":cluster{"OverlayEnable":bool, "OverlayText":string, "OverlayCoords":i32[], "OverlayAngle":dbl, "OverlayTextSize":dbl, "OverlayTextColor":string}, "ResultVariable":string}, "ROI2":cluster{"ROI":cluster{"Left":dbl, "Top":dbl, "Right":dbl, "Bottom":dbl, "Rotation":dbl}, "EdgeOptions":cluster{"EdgePoarity":dbl, "KernelSize":dbl, "Width":dbl, "MinimumEdgeStrength":dbl, "InterpolationType":dbl, "DataProcessingMethod":dbl}, "LineOptions":cluster{"NumberofLines":dbl, "Type":dbl, "MinScore":dbl, "MaxScore":dbl, "Orientation":dbl, "AngleRange":dbl, "AngleTolerance":dbl, "StepSize":dbl, "MinSNR":dbl, "MinPoints":dbl, "HoughIterations":dbl}, "Process":dbl, "StepSize":dbl, "SearchDirection":dbl, "CircleEdgeOptions":cluster{"SearchDirection":dbl, "EdgeOptions":cluster{"EdgePoarity":dbl, "KernelSize":dbl, "Width":dbl, "MinimumEdgeStrength":dbl, "InterpolationType":dbl, "DataProcessingMethod":dbl}}, "CircleFitOptions":cluster{"Process":dbl, "StepSize":dbl, "MaxPixelRadius":dbl}, "CircleSearchDirection":dbl, "CurveParameters":cluster{"ExtractionMode":dbl, "EdgeThreshold":dbl, "EdgeFilterSize":dbl, "MinLength":dbl, "RowSearchStepSize":dbl, "ColSearchStepSize":dbl, "MaxEndpointGap":dbl, "Closed":dbl, "Subpixel":dbl}, "MinimumMatchScore":dbl, "CircleDescriptor":cluster{"MinRadius":dbl, "MaxRadius":dbl}, "EllipseDescriptor":cluster{"MinMajorRadius":dbl, "MaxMajorRadius":dbl, "MinMinorRadius":dbl, "MaxMinorRadius":dbl}, "OverlayOptions":cluster{"OverlayEnable":bool, "OverlayText":string, "OverlayCoords":i32[], "OverlayAngle":dbl, "OverlayTextSize":dbl, "OverlayTextColor":string}, "ResultVariable":string}}, "MathExpressionDefault":cluster{"Algorithm":string, "MathExpression":string, "ResultVariable":string}}, "CalibrationCoefficients":cluster{"A1":dbl, "A2":dbl, "A3":dbl}, "UserCalibCoefficients":cluster{"UserCorrectionBiasCoeff":dbl, "UserCorrectionLinearityCoeff":dbl}, "OverlayOptions":cluster{"OverlayEnable":bool, "OverlayText":string, "OverlayCoords":i32[], "OverlayAngle":dbl, "OverlayTextSize":dbl, "OverlayTextColor":string}, "DatalogEnable":bool, "DisplayIcon":string}}
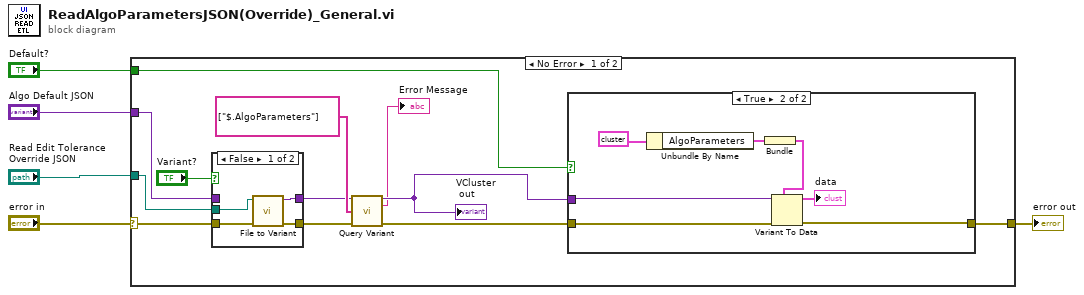
[diagram p0: block diagram]
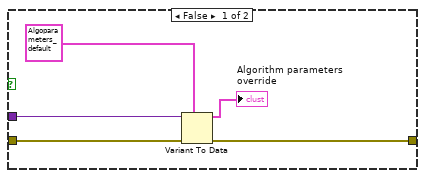
[diagram p2: hidden frame]
diagram:
  n1 = case shown="No Error" "error in" {
    selector: "error in" -> [w14 w36]
    tunnel: [w16 w36] -> w5
    tunnel: "Read Edit Tolerance \nOverride JSON" -> [w13 _]
    tunnel: "Algo Default JSON" -> [w9 _]
    tunnel: "Default?" -> [w6 _]
    frame No Error {
      n2 = case shown="False" "Variant?" {
        tunnel: w14 -> [w33 w35]
        tunnel: w13 -> [w31 _]
        tunnel: [w30 w34] -> w11
        tunnel: [w32 w35] -> w10
        tunnel: w9 -> [_ w34]
        frame False {
          n3 = call <vilib>:"File to Variant.vi"("JSON FilePath"=w31, "error in (no error)"=w33) -> ("JSON Variant"=w30:variant, "error out"=w32:errorcluster)  [unwired: 6 in, 1 out]
        }
        frame True {
        }
      }
      n4 = call <vilib>:"Query Variant.vi"("VCluster in"=w11, "pathList"=string[] ["$.AlgoParameters"], "error IO"=w10) -> ("VCluster\n out"=w17:variant, "Error Message"=→"Error Message":string, "error out"=w7:errorcluster)  [unwired: 9 in, 1 out]
      "VCluster\n out" <- w17
      n5 = case shown="True" w6 {
        tunnel: w17 -> [w22 w27]
        tunnel: [w21 w28] -> w16
        tunnel: w7 -> [w20 w29]
        frame False {
          n6 = Variant To Data(error in=w20, type=T2 {"AlgoParameters"={"PartsList"=[], "AlgoDefaultParameters"={"AlgoName"="", "Enable"=FALSE, "AlgorithmSequenceDefault"={"RefernceEdgeDefault"={"Method"="", "RefROI"={"Left"=0.0, "Top"=0.0, "Right"=0.0, "Bottom"=0.0, "Rotation"=0.0}, "EdgeOptions"={"EdgePoarity"=0.0, "KernelSize"=0.0, "Width"=0.0, "MinimumEdgeStrength"=0.0, "InterpolationType"=0.0, "DataProcessingMethod"=0.0}, "LineOptions"={"NumberofLines"=0.0, "Type"=0.0, "MinScore"=0.0, "MaxScore"=0.0, "Orientation"=0.0, "AngleRange"=0.0, "AngleTolerance"=0.0, "StepSize"=0.0, "MinSNR"=0.0, "MinPoints"=0.0, "HoughIterations"=0.0}, "SearchDirection"=0.0}, "MeasurementDefault"={"ROI1"={"ROI"={"Left"=0.0, "Top"=0.0, "Right"=0.0, "Bottom"=0.0, "Rotation"=0.0}, "EdgeOptions"={"EdgePoarity"=0.0, "KernelSize"=0.0, "Width"=0.0, "MinimumEdgeStrength"=0.0, "InterpolationType"=0.0, "DataProcessingMethod"=0.0}, "LineOptions"={"NumberofLines"=0.0, "Type"=0.0, "MinScore"=0.0, "MaxScore"=0.0, "Orientation"=0.0, "AngleRange"=0.0, "AngleTolerance"=0.0, "StepSize"=0.0, "MinSNR"=0.0, "MinPoints"=0.0, "HoughIterations"=0.0}, "Process"=0.0, "StepSize"=0.0, "SearchDirection"=0.0, "CircleEdgeOptions"={"SearchDirection"=0.0, "EdgeOptions"={"EdgePoarity"=0.0, "KernelSize"=0.0, "Width"=0.0, "MinimumEdgeStrength"=0.0, "InterpolationType"=0.0, "DataProcessingMethod"=0.0}}, "CircleFitOptions"={"Process"=0.0, "StepSize"=0.0, "MAxPixelRadius"=0.0}, "CircleSearchDirection"=0.0, "CurveParameters"={"ExtractionMode"=0.0, "EdgeThreshold"=0.0, "EdgeFilterSize"=0.0, "MinLength"=0.0, "RowSearchStepSize"=0.0, "ColSearchStepSize"=0.0, "MaxEndpointGap"=0.0, "Closed"=0.0, "Subpixel"=0.0}, "MinimumMatchScore"=0.0, "CircleDescriptor"={"MinRadius"=0.0, "MaxRadius"=0.0}, "EllipseDescriptor"={"MinMajorRadius"=0.0, "MaxMajorRadius"=0.0, "MinMinorRadius"=0.0, "MaxMinorRadius"=0.0}, "OverlayOptions"={"OverlayEnable"=FALSE, "OverlayText"="", "OverlayCoords"=[], "OverlayAngle"=0.0, "OverlayTextSize"=0.0, "OverlayTextColor"=""}, "ResultVariable"=""}, "ROI2"={"ROI"={"Left"=0.0, "Top"=0.0, "Right"=0.0, "Bottom"=0.0, "Rotation"=0.0}, "EdgeOptions"={"EdgePoarity"=0.0, "KernelSize"=0.0, "Width"=0.0, "MinimumEdgeStrength"=0.0, "InterpolationType"=0.0, "DataProcessingMethod"=0.0}, "LineOptions"={"NumberofLines"=0.0, "Type"=0.0, "MinScore"=0.0, "MaxScore"=0.0, "Orientation"=0.0, "AngleRange"=0.0, "AngleTolerance"=0.0, "StepSize"=0.0, "MinSNR"=0.0, "MinPoints"=0.0, "HoughIterations"=0.0}, "Process"=0.0, "StepSize"=0.0, "SearchDirection"=0.0, "CircleEdgeOptions"={"SearchDirection"=0.0, "EdgeOptions"={"EdgePoarity"=0.0, "KernelSize"=0.0, "Width"=0.0, "MinimumEdgeStrength"=0.0, "InterpolationType"=0.0, "DataProcessingMethod"=0.0}}, "CircleFitOptions"={"Process"=0.0, "StepSize"=0.0, "MaxPixelRadius"=0.0}, "CircleSearchDirection"=0.0, "CurveParameters"={"ExtractionMode"=0.0, "EdgeThreshold"=0.0, "EdgeFilterSize"=0.0, "MinLength"=0.0, "RowSearchStepSize"=0.0, "ColSearchStepSize"=0.0, "MaxEndpointGap"=0.0, "Closed"=0.0, "Subpixel"=0.0}, "MinimumMatchScore"=0.0, "CircleDescriptor"={"MinRadius"=0.0, "MaxRadius"=0.0}, "EllipseDescriptor"={"MinMajorRadius"=0.0, "MaxMajorRadius"=0.0, "MinMinorRadius"=0.0, "MaxMinorRadius"=0.0}, "OverlayOptions"={"OverlayEnable"=FALSE, "OverlayText"="", "OverlayCoords"=[], "OverlayAngle"=0.0, "OverlayTextSize"=0.0, "OverlayTextColor"=""}, "ResultVariable"=""}}, "MathExpressionDefault"={"Algorithm"="", "MathExpression"="", "ResultVariable"=""}}, "CalibrationCoefficients"={"A1"=0.0, "A2"=0.0, "A3"=0.0}, "UserCalibCoefficients"={"UserCorrectionBiasCoeff"=0.0, "UserCorrectionLinearityCoeff"=0.0}, "OverlayOptions"={"OverlayEnable"=FALSE, "OverlayText"="", "OverlayCoords"=[], "OverlayAngle"=0.0, "OverlayTextSize"=0.0, "OverlayTextColor"=""}, "DatalogEnable"=FALSE, "DisplayIcon"=""}}}, Variant=w22) -> (data=→"Algorithm parameters\noverride":T2, error out=w21:errorcluster)
        }
        frame True {
          n7 = Unbundle By Name(T3 {"SpecificationVersion"="", "CompatibleSoftwareVersions"=[], "AlgoParameters"={"PartsList"=[], "AlgoDefaultParameters"={"AlgoName"="", "Enable"=FALSE, "AlgorithmSequenceDefault"={"RefernceEdgeDefault"={"Method"="", "RefROI"={"Left"=0.0, "Top"=0.0, "Right"=0.0, "Bottom"=0.0, "Rotation"=0.0}, "EdgeOptions"={"EdgePoarity"=0.0, "KernelSize"=0.0, "Width"=0.0, "MinimumEdgeStrength"=0.0, "InterpolationType"=0.0, "DataProcessingMethod"=0.0}, "LineOptions"={"NumberofLines"=0.0, "Type"=0.0, "MinScore"=0.0, "MaxScore"=0.0, "Orientation"=0.0, "AngleRange"=0.0, "AngleTolerance"=0.0, "StepSize"=0.0, "MinSNR"=0.0, "MinPoints"=0.0, "HoughIterations"=0.0}, "SearchDirection"=0.0}, "MeasurementDefault"={"ROI1"={"ROI"={"Left"=0.0, "Top"=0.0, "Right"=0.0, "Bottom"=0.0, "Rotation"=0.0}, "EdgeOptions"={"EdgePoarity"=0.0, "KernelSize"=0.0, "Width"=0.0, "MinimumEdgeStrength"=0.0, "InterpolationType"=0.0, "DataProcessingMethod"=0.0}, "LineOptions"={"NumberofLines"=0.0, "Type"=0.0, "MinScore"=0.0, "MaxScore"=0.0, "Orientation"=0.0, "AngleRange"=0.0, "AngleTolerance"=0.0, "StepSize"=0.0, "MinSNR"=0.0, "MinPoints"=0.0, "HoughIterations"=0.0}, "Process"=0.0, "StepSize"=0.0, "SearchDirection"=0.0, "CircleEdgeOptions"={"SearchDirection"=0.0, "EdgeOptions"={"EdgePoarity"=0.0, "KernelSize"=0.0, "Width"=0.0, "MinimumEdgeStrength"=0.0, "InterpolationType"=0.0, "DataProcessingMethod"=0.0}}, "CircleFitOptions"={"Process"=0.0, "StepSize"=0.0, "MAxPixelRadius"=0.0}, "CircleSearchDirection"=0.0, "CurveParameters"={"ExtractionMode"=0.0, "EdgeThreshold"=0.0, "EdgeFilterSize"=0.0, "MinLength"=0.0, "RowSearchStepSize"=0.0, "ColSearchStepSize"=0.0, "MaxEndpointGap"=0.0, "Closed"=0.0, "Subpixel"=0.0}, "MinimumMatchScore"=0.0, "CircleDescriptor"={"MinRadius"=0.0, "MaxRadius"=0.0}, "EllipseDescriptor"={"MinMajorRadius"=0.0, "MaxMajorRadius"=0.0, "MinMinorRadius"=0.0, "MaxMinorRadius"=0.0}, "OverlayOptions"={"OverlayEnable"=FALSE, "OverlayText"="", "OverlayCoords"=[], "OverlayAngle"=0.0, "OverlayTextSize"=0.0, "OverlayTextColor"=""}, "ResultVariable"=""}, "ROI2"={"ROI"={"Left"=0.0, "Top"=0.0, "Right"=0.0, "Bottom"=0.0, "Rotation"=0.0}, "EdgeOptions"={"EdgePoarity"=0.0, "KernelSize"=0.0, "Width"=0.0, "MinimumEdgeStrength"=0.0, "InterpolationType"=0.0, "DataProcessingMethod"=0.0}, "LineOptions"={"NumberofLines"=0.0, "Type"=0.0, "MinScore"=0.0, "MaxScore"=0.0, "Orientation"=0.0, "AngleRange"=0.0, "AngleTolerance"=0.0, "StepSize"=0.0, "MinSNR"=0.0, "MinPoints"=0.0, "HoughIterations"=0.0}, "Process"=0.0, "StepSize"=0.0, "SearchDirection"=0.0, "CircleEdgeOptions"={"SearchDirection"=0.0, "EdgeOptions"={"EdgePoarity"=0.0, "KernelSize"=0.0, "Width"=0.0, "MinimumEdgeStrength"=0.0, "InterpolationType"=0.0, "DataProcessingMethod"=0.0}}, "CircleFitOptions"={"Process"=0.0, "StepSize"=0.0, "MaxPixelRadius"=0.0}, "CircleSearchDirection"=0.0, "CurveParameters"={"ExtractionMode"=0.0, "EdgeThreshold"=0.0, "EdgeFilterSize"=0.0, "MinLength"=0.0, "RowSearchStepSize"=0.0, "ColSearchStepSize"=0.0, "MaxEndpointGap"=0.0, "Closed"=0.0, "Subpixel"=0.0}, "MinimumMatchScore"=0.0, "CircleDescriptor"={"MinRadius"=0.0, "MaxRadius"=0.0}, "EllipseDescriptor"={"MinMajorRadius"=0.0, "MaxMajorRadius"=0.0, "MinMinorRadius"=0.0, "MaxMinorRadius"=0.0}, "OverlayOptions"={"OverlayEnable"=FALSE, "OverlayText"="", "OverlayCoords"=[], "OverlayAngle"=0.0, "OverlayTextSize"=0.0, "OverlayTextColor"=""}, "ResultVariable"=""}}, "MathExpressionDefault"={"Algorithm"="", "MathExpression"="", "ResultVariable"=""}}, "CalibrationCoefficients"={"A1"=0.0, "A2"=0.0, "A3"=0.0}, "UserCalibCoefficients"={"UserCorrectionBiasCoeff"=0.0, "UserCorrectionLinearityCoeff"=0.0}, "OverlayOptions"={"OverlayEnable"=FALSE, "OverlayText"="", "OverlayCoords"=[], "OverlayAngle"=0.0, "OverlayTextSize"=0.0, "OverlayTextColor"=""}, "DatalogEnable"=FALSE, "DisplayIcon"=""}}} ("AlgoParameters_default")) -> ("AlgoParameters"=w25:T4)
          n8 = Bundle("AlgoParameters"=w25) -> (w24:T1)  [unwired: 1 in]
          n9 = Variant To Data(error in=w29, type=w24, Variant=w27) -> (data=→"data":T1, error out=w28:errorcluster)
        }
      }
    }
    frame Error {
    }
  }
  "error out" <- w5
